vi "Obtain Broadcast Events.vi"(8 "error in (no error)":errorcluster, 10 "Create New?":bool) -> (0 "error out":errorcluster, 2 "UI Manager Broadcast Events":T1)   [LabVIEW 2022 SP3, in "UI Manager.lvlib"]
doc: "This VI Obtains/Creates the Broadcast events that will be used for other modules to register to receive messages from the module that owns this VI.\n\n<b>NOTE</b>: The contents of this VI are automatically generated and modified by the <b>Tools > Delacor > DQMH</b> utilities. Consider using those utilities instead of making your own modifications to this VI.\n____\nHAMPEL SOFTWARE ENGINEERING v2.6.0 (2023-12-19 10:54)"
uses:
  UI Manager.lvlib
  Broadcast Events--cluster.ctl
  Did Init Argument--cluster.ctl
  Status Updated Argument--cluster.ctl
  Error Reported Argument--cluster.ctl
  Stop Argument--cluster.ctl
  Get Module Execution Status Argument--cluster.ctl
  System Message Argument--cluster.ctl
  Libraries/hse-libraries/Source/hse-dqmh/Controls/System Message Source.ctl
  Login Argument--cluster.ctl
  Key down Argument--cluster.ctl
  <vilib>/event_ctls.llb/eventvkey.ctl
  Libraries/hse-libraries/Source/hse-dqmh/hse-dqmh.lvlib
panel:
  # "NOTE: The contents of this VI are automatically generated and modified by the Tools > Delacor > DQMH utilities. Consider using those utilities instead of making your own modifications to this VI."
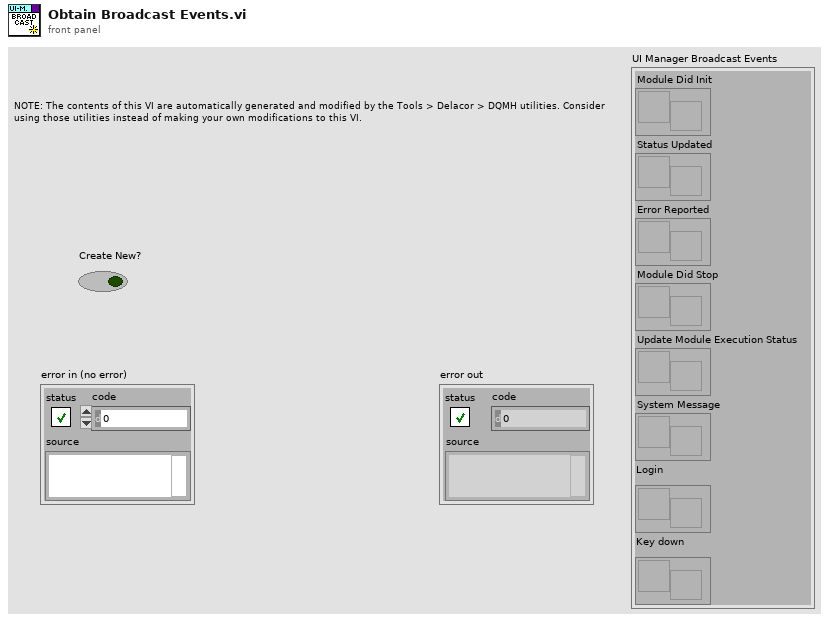
[diagram p1: front panel]
types:
  T1 = typedef "UI Manager.lvlib/Broadcast Events--cluster.ctl" = cluster{"Module Did Init":refnum<user-event>, "Status Updated":refnum<user-event>, "Error Reported":refnum<user-event>, "Module Did Stop":refnum<user-event>, "Update Module Execution Status":refnum<user-event>, "System Message":refnum<user-event>, "Login":refnum<user-event>, "Key down":refnum<user-event>}
  T2 = typedef "UI Manager.lvlib/Key down Argument--cluster.ctl" = cluster{"VKey":T3, "Char":i16, "PlatMods":cluster{"Shift":bool, "Ctrl":bool, "Alt":bool, "Cmd":bool, "Opt":bool}}
  T3 = typedef "eventvkey.ctl" = enum16{"ASCII", "Enter", "Return", "Shift", "Ctrl", "Alt", "Cmd", "Opt", "Caps", "NumLock", "Clear", "Break", "Up", "Down", "Left", "Right", "Insert", "Delete", "Home", "End", "PageUp", "PageDown", "Escape", "Help", "Pause", "ScrollLock", "F1", "F2", "F3", "F4", "F5", "F6", "F7", "F8", "F9", "F10", "F11", "F12", "F13", "F14", "F15", "F16", "F17", "F18", "F19", "F20", "F21", "F22", "F23", "F24", "Play", "VolumeUp", "VolumeDown", "Mute", "Two Byte Char"}
  T4 = typedef "UI Manager.lvlib/Login Argument--cluster.ctl" = cluster{"User Name":string, "User Level":string}
  T5 = typedef "UI Manager.lvlib/System Message Argument--cluster.ctl" = cluster{"Identifier":string, "Payload":variant, "Sys. Msg. Source":T6, "Sys. Msg. Origin":string}
  T6 = typedef "hse-dqmh.lvlib/System Message Source.ctl" = enum16{"module", "application", "network"}
  T7 = typedef "UI Manager.lvlib/Get Module Execution Status Argument--cluster.ctl" = cluster{"Running?":bool}
  T8 = typedef "UI Manager.lvlib/Stop Argument--cluster.ctl" = cluster{"Origin":string, "Exit via Stop Module Req?":bool, "Wait for Module to stop?":bool}
  T9 = typedef "UI Manager.lvlib/Error Reported Argument--cluster.ctl" = cluster{"Error":errorcluster, "Additional Information":string, "Module Name":string}
  T10 = typedef "UI Manager.lvlib/Status Updated Argument--cluster.ctl" = cluster{"Status":string}
  T11 = typedef "UI Manager.lvlib/Did Init Argument--cluster.ctl" = cluster{"Init?":bool, "Info":string}
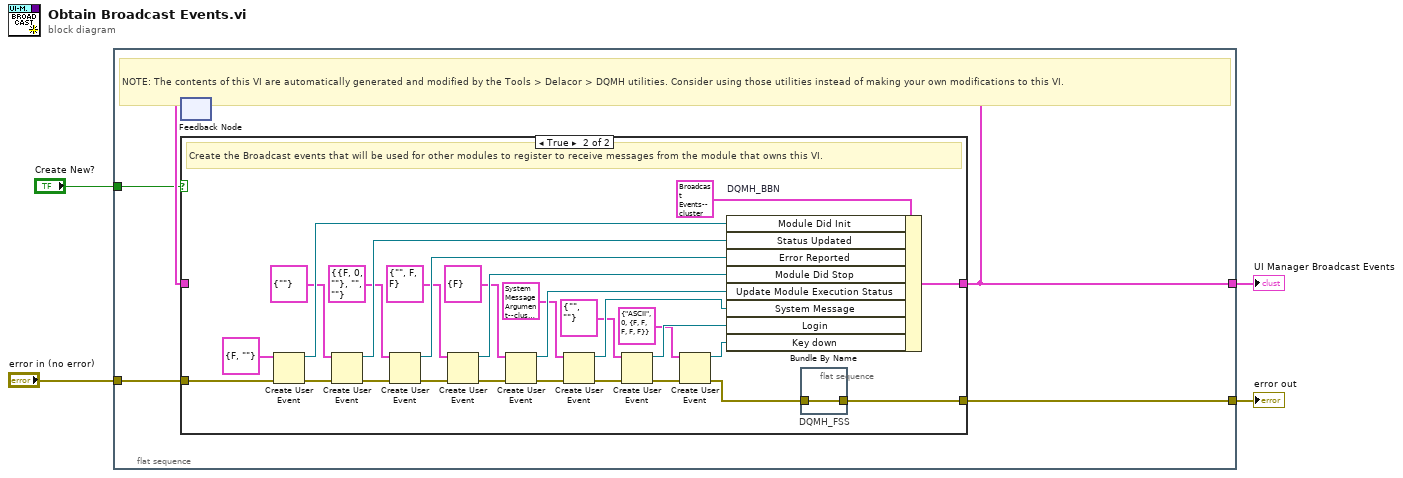
[diagram p0: block diagram]
diagram:
  n1 = flat-sequence {
    tunnel: [w9] -> w4
    tunnel: "error in (no error)" -> [w8]
    tunnel: [w6] -> w2
    tunnel: "Create New?" -> [w5]
    frame #0 {
      # "NOTE: The contents of this VI are automatically generated and modified by the Tools > Delacor > DQMH utilities. Consider using those utilities instead of making your own modifications to this VI."
      n2 = feedback #1() -> (w7:T1)  [unwired: 1 in]
      n3 = case shown="True" w5 {
        tunnel: [w10 w24] -> w9
        tunnel: w8 -> [w10 w39]
        tunnel: [w11 w36] -> w6
        tunnel: w7 -> [w11 _]
        frame False {
          # "Obtain the Broadcast events that were created in a previous call to this VI."
        }
        frame True {
          # "Create the Broadcast events that will be used for other modules to register to receive messages from the module that owns this VI."
          n4 = Create User Event(user event datatype=T11 {"Init?"=FALSE, "Info"=""} ("Did Init Argument"), error in=w39) -> (user event=w37:refnum<user-event>, error out=w34:errorcluster)
          n5 = Create User Event(user event datatype=T10 {"Status"=""} ("Status Updated Argument"), error in=w34) -> (user event=w31:refnum<user-event>, error out=w33:errorcluster)
          n6 = Create User Event(user event datatype=T9 {"Error"={"status"=FALSE, "code"=0, "source"=""}, "Additional Information"="", "Module Name"=""} ("Error Reported Argument"), error in=w33) -> (user event=w28:refnum<user-event>, error out=w30:errorcluster)
          n7 = Create User Event(user event datatype=T8 {"Origin"="", "Exit via Stop Module Req?"=FALSE, "Wait for Module to stop?"=FALSE} ("Stop Argument"), error in=w30) -> (user event=w26:refnum<user-event>, error out=w25:errorcluster)
          n8 = Create User Event(user event datatype=T7 {"Running?"=FALSE} ("Get Module Execution Status Argument"), error in=w25) -> (user event=w22:refnum<user-event>, error out=w23:errorcluster)
          n9 = Create User Event(user event datatype=T5 {"Identifier"="", "Payload"=variant, "Sys. Msg. Source"=enum."module", "Sys. Msg. Origin"=""} ("System Message Argument"), error in=w23) -> (user event=w19:refnum<user-event>, error out=w20:errorcluster)
          n10 = Create User Event(user event datatype=T4 {"User Name"="", "User Level"=""} ("Login Argument"), error in=w20) -> (user event=w16:refnum<user-event>, error out=w17:errorcluster)
          n11 = Create User Event(user event datatype=T2 {"VKey"=enum."ASCII", "Char"=0, "PlatMods"={"Shift"=FALSE, "Ctrl"=FALSE, "Alt"=FALSE, "Cmd"=FALSE, "Opt"=FALSE}} ("Key down Argument"), error in=w17) -> (user event=w13:refnum<user-event>, error out=w14:errorcluster)
          n12 = Bundle By Name "DQMH_BBN"(cluster=T1 {"Module Did Init"=refnum, "Status Updated"=refnum, "Error Reported"=refnum, "Module Did Stop"=refnum, "Update Module Execution Status"=refnum, "System Message"=refnum, "Login"=refnum, "Key down"=refnum} ("output cluster"), "Module Did Init"=w37, "Status Updated"=w31, "Error Reported"=w28, "Module Did Stop"=w26, "Update Module Execution Status"=w22, "System Message"=w19, "Login"=w16, "Key down"=w13) -> (w36:T1)
          n13 = flat-sequence "DQMH_FSS" {
            tunnel: w14 -> [w40]
            tunnel: [w40] -> w24
            frame #0 {
            }
          }
        }
      }
      n14 = feedback-in #1(w6) -> ()
    }
  }
  "UI Manager Broadcast Events" <- w2
  "error out" <- w4
